vi "AlliGator Get Image & FLI Dataset Paths.vi"(8 "error in (no error)":errorcluster, 10 "File names":string[](array[string]), 11 "Directory path":path) -> (0 "error out":errorcluster, 2 "FLI Dataset Paths":path[](array[path]), 3 "Image Paths":path[](array[path]))   [LabVIEW 2021, in "AlliGator Files.lvlib"]
doc: "Gets FLI dataset paths (or image paths if the files are of that type)."
uses:
  AlliGator Files.lvlib
  Image/Image.lvlib
panel:
  # "see the AlliGator License on the block diagram (Ctrl+E or Window:Show Block Diagram)"
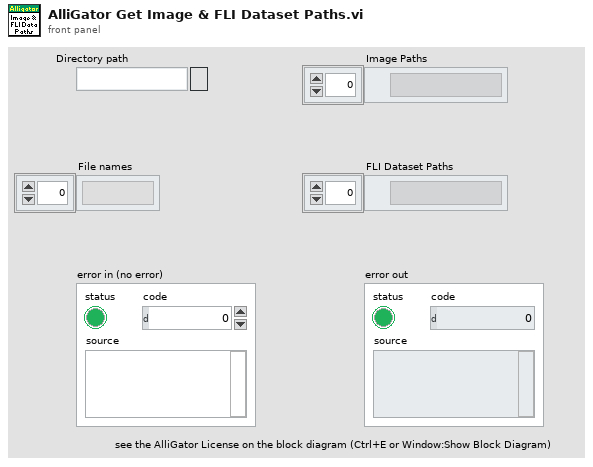
[diagram p1: front panel]
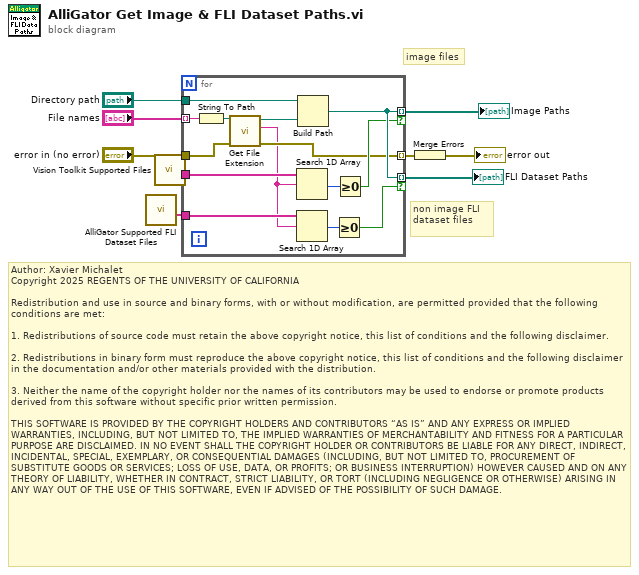
[diagram p0: block diagram]
diagram:
  # "Author: Xavier Michalet\nCopyright 2025 REGENTS OF THE UNIVERSITY OF CALIFORNIA\n\nRedistribution and use in source and binary forms, with or without modification, are permitted provided that the following conditions are met:\n\n1. Redistributions of source code must retain the above copyright notice, this list of conditions and the following disclaimer.\n\n2. Redistributions in binary form must reproduce the above copyright notice, this list of conditions and the following disclaimer in the documentation and/or other materials provided with the distribution.\n\n3. Neither the name of the copyright holder nor the names of its contributors may be used to endorse or promote products derived from this software without specific prior written permission.\n\nTHIS SOFTWARE IS PROVIDED BY THE COPYRIGHT HOLDERS AND CONTRIBUTORS “AS IS” AND ANY EXPRESS OR IMPLIED WARRANTIES, INCLUDING, BUT NOT LIMITED TO, THE IMPLIED WARRANTIES OF MERCHANTABILITY AND FITNESS FOR A PARTICULAR PURPOSE ARE DISCLAIMED. IN NO EVENT SHALL THE COPYRIGHT HOLDER OR CONTRIBUTORS BE LIABLE FOR ANY DIRECT, INDIRECT, INCIDENTAL, SPECIAL, EXEMPLARY, OR CONSEQUENTIAL DAMAGES (INCLUDING, BUT NOT LIMITED TO, PROCUREMENT OF SUBSTITUTE GOODS OR SERVICES; LOSS OF USE, DATA, OR PROFITS; OR BUSINESS INTERRUPTION) HOWEVER CAUSED AND ON ANY THEORY OF LIABILITY, WHETHER IN CONTRACT, STRICT LIABILITY, OR TORT (INCLUDING NEGLIGENCE OR OTHERWISE) ARISING IN ANY WAY OUT OF THE USE OF THIS SOFTWARE, EVEN IF ADVISED OF THE POSSIBILITY OF SUCH DAMAGE."
  # "non image FLI dataset files"
  # "image files"
  n1 = call "AlliGator Supported FLI Dataset Files.vi"() -> ("File Extensions"=w6:string[])  [unwired: 7 in, 1 out]
  n2 = call "Vision Toolkit Supported Files.vi"() -> ("File Extensions"=w5:string[])  [unwired: 7 in, 1 out]
  n3 = for {
    tunnel: "File names" -> [w23] mode=indexing
    tunnel: "error in (no error)" -> [w21]
    tunnel: w5 -> [w20]
    tunnel: "Directory path" -> [w19]
    tunnel: [w16] -> w7 mode=indexing if=w15
    tunnel: [w16] -> w8 mode=indexing if=w10
    tunnel: [w14] -> w3 mode=indexing
    tunnel: w6 -> [w13]
    n4 = String To Path(string=w23) -> (path=w22:path)
    n5 = call <vilib>:"Get File Extension.vi"("error in (no error)"=w21, "file"=w22) -> ("error out"=w14:errorcluster, "lowercase file extension"=w12:string, "dup file"=w18:path)  [unwired: 5 in, 2 out]
    n6 = Search 1D Array(1D array=w20, element=w12) -> (index of element=w17:i32)  [unwired: 1 in]
    n7 = Search 1D Array(1D array=w13, element=w12) -> (index of element=w11:i32)  [unwired: 1 in]
    n8 = Build Path(base path=w19, name or relative path=w18) -> (appended path=w16:path)
    n9 = Greater Or Equal To 0?(x=w11) -> (x >= 0?=w10:bool)
    n10 = Greater Or Equal To 0?(x=w17) -> (x >= 0?=w15:bool)
  }
  "FLI Dataset Paths" <- w8
  "Image Paths" <- w7
  n11 = Merge Errors(w3) -> (→"error out":errorcluster)
